vi "SubVI_Draw Point #.vi"(4 "Color":u32(colorbox)=6618880, 5 "Group":string, 6 "error in":errorcluster, 7 "Radius":i32=4, 8 "Points":cluster{"X":i32, "Y":i32}[](array[cluster]), 9 "Image In":T1) -> (0 "error out":errorcluster, 3 "Image Out":T1)   [LabVIEW 2013]
uses:
  <vilib>/vision/Image Controls.llb/IMAQ Image.ctl
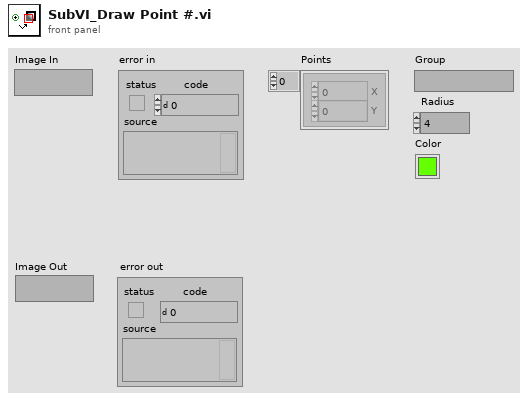
[diagram p1: front panel]
types:
  T1 = typedef "IMAQ Image.ctl" = refnum<image>
  T2 = cluster{"Left":i32, "Top":i32, "Right":i32, "Bottom":i32}
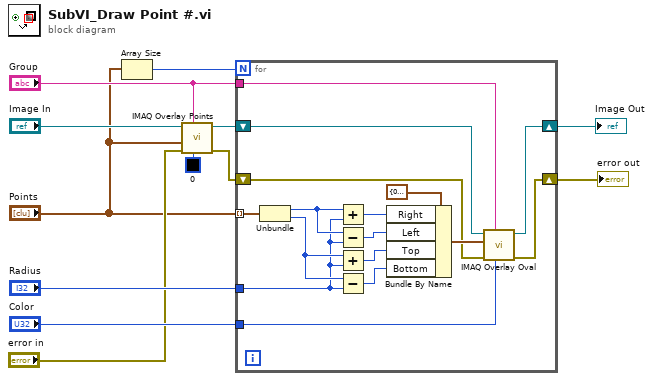
[diagram p0: block diagram]
diagram:
  n1 = Array Size(array="Points") -> (size(s)=w1:i32)
  n2 = call "IMAQ Overlay Points"("Color"=u32 0, "Group"="Group", "error in (no error)"="error in", "Array of Points"="Points", "Image"="Image In") -> ("error out"=w6:errorcluster, "Image Out"=w7:T1)  [unwired: 5 in]
  n3 = for {
    N: w1 -> [_]
    tunnel: "Points" -> [w28] mode=indexing
    tunnel: "Radius" -> [w25]
    tunnel: "Color" -> [w18]
    shift-right: [w17] -> w8
    shift-left: w7 -> [w16]
    tunnel: "Group" -> [w15]
    shift-right: [w13] -> w3
    shift-left: w6 -> [w14]
    n4 = Unbundle(w28) -> ("X"=w27:i32, "Y"=w26:i32)
    n5 = Add(x=w27, y=w25) -> (x+y=w23:i32)
    n6 = Subtract(x=w27, y=w25) -> (x-y=w22:i32)
    n7 = Add(x=w26, y=w25) -> (x+y=w21:i32)
    n8 = Subtract(x=w26, y=w25) -> (x-y=w20:i32)
    n9 = Bundle By Name(cluster=T2 {"Left"=0, "Top"=0, "Right"=0, "Bottom"=0} ("Bounding Rectangle"), "Right"=w23, "Left"=w22, "Top"=w21, "Bottom"=w20) -> (w19:T2)
    n10 = call "IMAQ Overlay Oval"("Color"=w18, "Group"=w15, "error in (no error)"=w14, "Bounding Rectangle"=w19, "Image"=w16) -> ("error out"=w13:errorcluster, "Image Out"=w17:T1)  [unwired: 5 in]
  }
  "Image Out" <- w8
  "error out" <- w3
